vi "parse.vi"(8 "error in (no error)":errorcluster, 9 "SwapBytes":bool, 10 "Data":u8[](array[numeric]), 11 "U8ArrayParserManualIndexing in":refnum<class "U8ArrayParserManualIndexing.lvclass">) -> (0 "error out":errorcluster, 3 "U8ArrayParserManualIndexing out":refnum<class "U8ArrayParserManualIndexing.lvclass">)   [LabVIEW 2016, in "RTUtilities.lvlib" / "U8ArrayParserManualIndexing.lvclass"]
uses:
  U8ArrayParserManualIndexing.lvclass
  U8ArrayParserManualIndexing.lvclass/U8ArrayParserManualIndexing.ctl
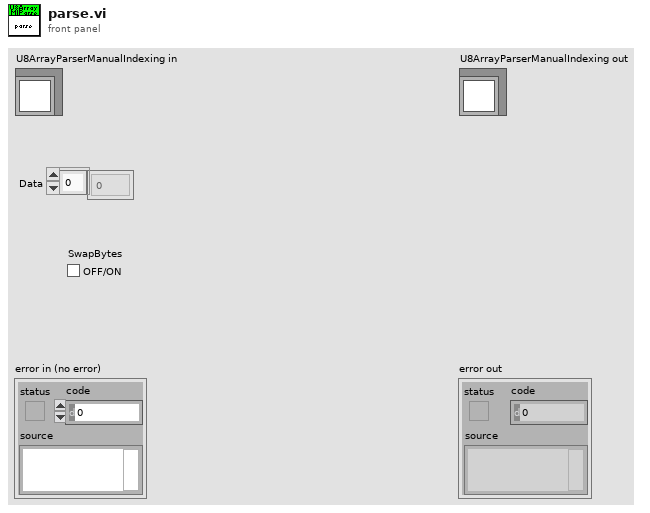
[diagram p1: front panel]
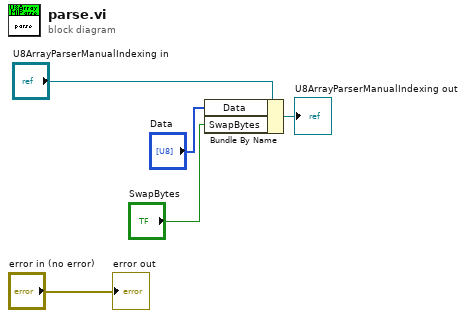
[diagram p0: block diagram]
diagram:
  n1 = Bundle By Name(cluster="U8ArrayParserManualIndexing in", "Data"="Data", "SwapBytes"="SwapBytes") -> (→"U8ArrayParserManualIndexing out":refnum<class "U8ArrayParserManualIndexing.lvclass">)
  "error out" <- "error in (no error)"
